vi "GetLabVIEWInfos.vi"(8 "error in (no error)":errorcluster, 11 "application.lvclass":refnum<class "application.lvclass">) -> (0 "error out":errorcluster, 3 "application.lvclass (dup)":refnum<class "application.lvclass">)   [LabVIEW 2017, in "application.lvlib" / "application.lvclass"]
uses:
  application.lvclass
  DEF-LabVIEW INFO.ctl
  application.lvclass/application.ctl
panel:
  out "LabVIEW Info":T1[](array[typedef])
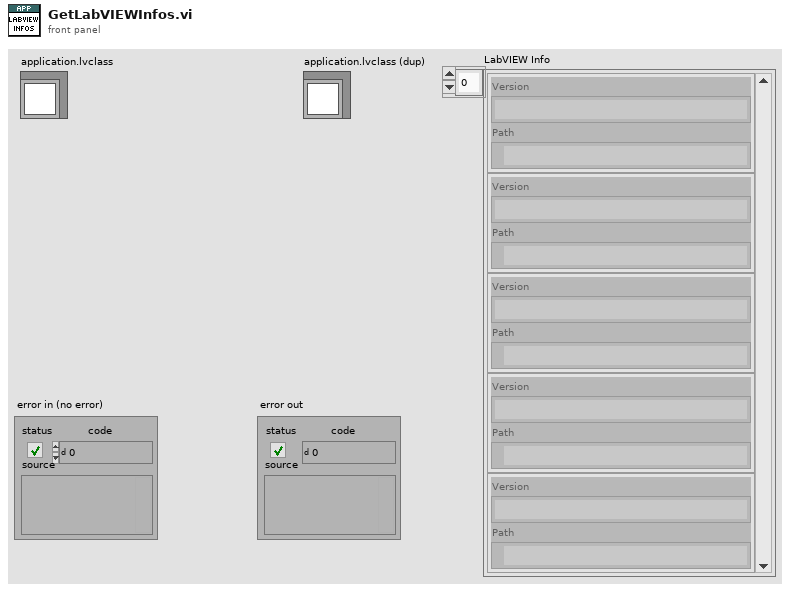
[diagram p1: front panel]
types:
  T1 = typedef "application.lvlib/application.lvclass/DEF-LabVIEW INFO.ctl" = cluster{"Version":string, "Path":path}
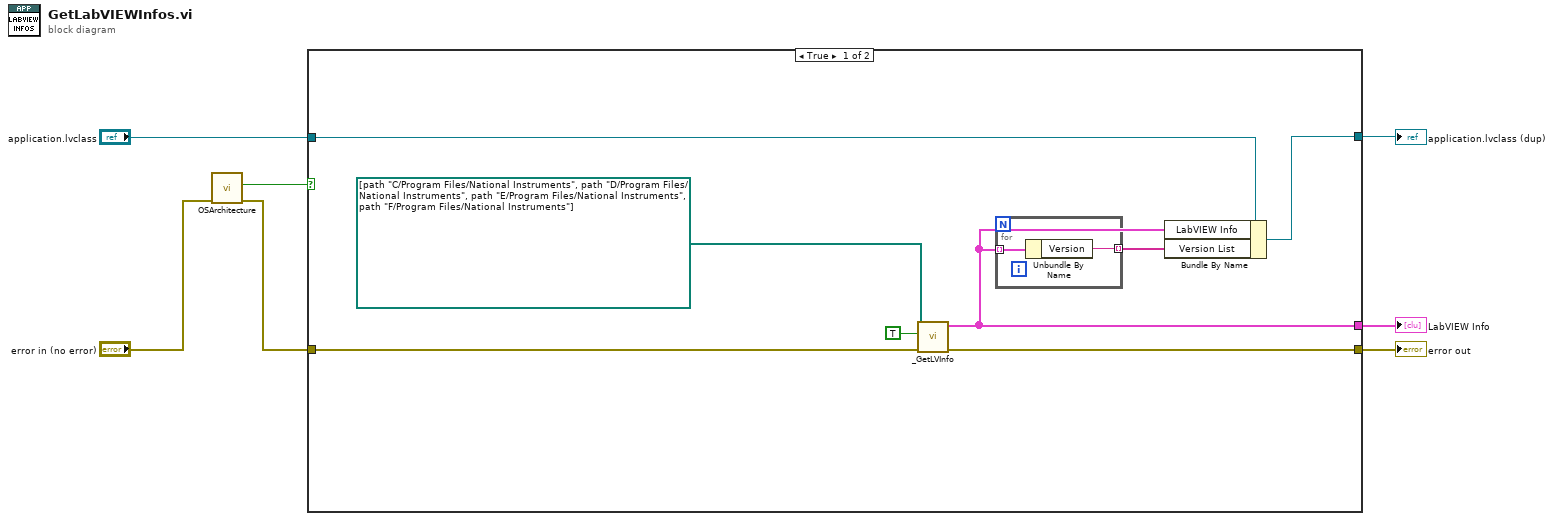
[diagram p0: block diagram]
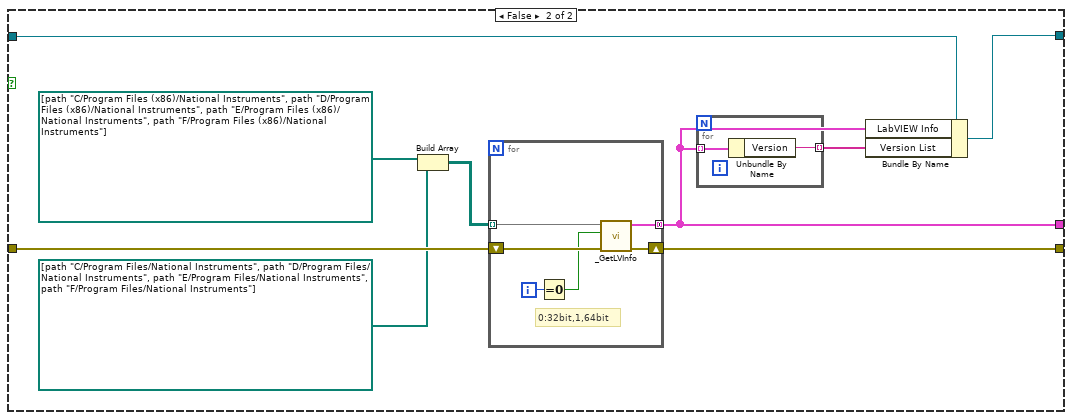
[diagram p2: hidden frame]
diagram:
  n1 = call "OSArchitecture.vi"("error in (no error)"="error in (no error)") -> ("error out"=w3:errorcluster, "32bit(T)/64bit(F)"=w2:bool)  [unwired: 9 in]
  n2 = case shown="True" w2 {
    tunnel: [w15 w26] -> w7
    tunnel: [w13 w24] -> w6
    tunnel: [w12 w23] -> w5
    tunnel: "application.lvclass" -> [w11 w22]
    tunnel: w3 -> [w10 w21]
    frame True {
      n3 = call "_GetLVInfo.vi"("error in (no error)"=w10, "32bit(T)/64bit(F)"=TRUE, "Array"=path[] [path "C:/Program Files/National Instruments", path "D:/Program Files/National Instruments", path "E:/Program Files/National Instruments", path "F:/Program Files/National Instruments"]) -> ("error out"=w15:errorcluster, "LabVIEW Info"=w13:T1[])  [unwired: 7 in]
      n4 = for {
        tunnel: w13 -> [w17] mode=indexing
        tunnel: [w16] -> w14 mode=indexing
        n5 = Unbundle By Name(w17) -> ("Version"=w16:string)
      }
      n6 = Bundle By Name(cluster=w11, "LabVIEW Info"=w13, "Version List"=w14) -> (w12:refnum<class "application.lvclass">)
    }
    frame False {
      n7 = Build Array(path[] [path "C:/Program Files (x86)/National Instruments", path "D:/Program Files (x86)/National Instruments", path "E:/Program Files (x86)/National Instruments", path "F:/Program Files (x86)/National Instruments"], path[] [path "C:/Program Files/National Instruments", path "D:/Program Files/National Instruments", path "E:/Program Files/National Instruments", path "F:/Program Files/National Instruments"]) -> (w18:path[][])
      n8 = for {
        tunnel: [w31] -> w24 mode=concatenating
        shift-right: [w32] -> w26
        shift-left: w21 -> [w30]
        tunnel: w18 -> [w29] mode=indexing
        i -> [w28]
        # "0:32bit,1,64bit"
        n9 = Equal To 0?(x=w28) -> (x = 0?=w27:bool)
        n10 = call "_GetLVInfo.vi"("error in (no error)"=w30, "32bit(T)/64bit(F)"=w27, "Array"=w29) -> ("error out"=w32:errorcluster, "LabVIEW Info"=w31:T1[])  [unwired: 7 in]
      }
      n11 = for {
        tunnel: w24 -> [w34] mode=indexing
        tunnel: [w33] -> w25 mode=indexing
        n12 = Unbundle By Name(w34) -> ("Version"=w33:string)
      }
      n13 = Bundle By Name(cluster=w22, "LabVIEW Info"=w24, "Version List"=w25) -> (w23:refnum<class "application.lvclass">)
    }
  }
  "LabVIEW Info" <- w6
  "error out" <- w7
  "application.lvclass (dup)" <- w5
